vi "OAT Truncate Speed Profile.vi"(9 "window info":T2={"window type"=10, "window length"=2048} {"window type" items=["None"=0, "Hanning"=1, "Hamming"=2, "Blackman-Harris"=3, "Exact Blackman"=4, "Blackman"=5, "Flat Top"=6, "4 Term B-Harris"=7, "7 Term B-Harris"=8, "Low Sidelobe"=9, "Gaussian"=62]; "window length" min=0}, 10 "speed profile 2":T1 {"speed [RPM]" format="%.2f"; "time [s]" format="%.2f"}, 11 "order waveforms [EU]":waveform(dbl)[](array[waveform])) -> (2 "speed profile":T1 {"speed [RPM]" format="%.2f"; "time [s]" format="%.2f"})   [LabVIEW 2017, in "SoundVib_Resampling.lvlib"]
uses:
  <vilib>/addons/Sound and Vibration/Order Analysis/Resample Order Tracking/SoundVib_Resampling.lvlib
  <vilib>/addons/Sound and Vibration/Order Analysis/Ref Gabor Order Tracking/window information.ctl
  <vilib>/addons/Sound and Vibration/Order Analysis/Tach Process/SubVIs/speed profile.ctl
  <vilib>/addons/Sound and Vibration/Order Analysis/Tach Process/SoundVib_TachProcess.lvlib
  <vilib>/addons/Sound and Vibration/Order Analysis/Gabor Order Tracking/SoundVib_Gabor.lvlib
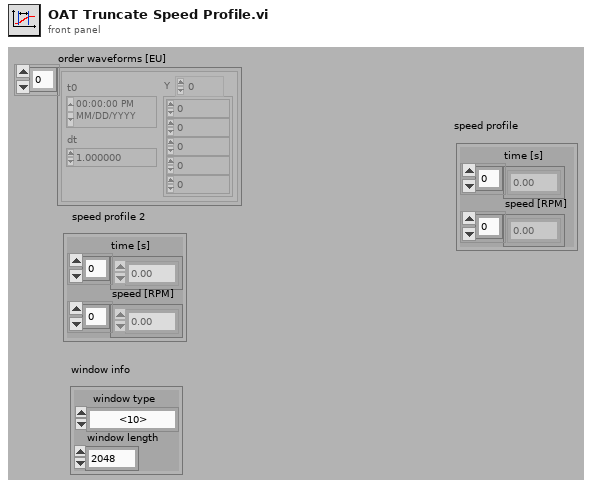
[diagram p1: front panel]
types:
  T1 = typedef "SoundVib_TachProcess.lvlib/speed profile.ctl" = cluster{"time [s]":dbl[], "speed [RPM]":dbl[]}
  T2 = typedef "SoundVib_Gabor.lvlib/window information.ctl" = cluster{"window type":u32, "window length":i32}
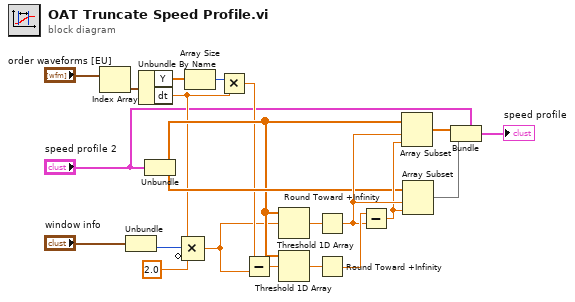
[diagram p0: block diagram]
diagram:
  n1 = Index Array(array="order waveforms [EU]") -> (element=w2:waveform(dbl))  [unwired: 1 in]
  n2 = Unbundle("window info") -> ("window length"=w11:i32)  [unwired: 1 out]
  n3 = Unbundle By Name(w2) -> ("Y"=w21:dbl[], "dt"=w8:dbl)
  n4 = Unbundle("speed profile 2") -> ("time [s]"=w12:dbl[], "speed [RPM]"=w17:dbl[])
  n5 = Compound Arithmetic op=MULTIPLY(w8, w11, invert 2.0) -> (w6:dbl)
  n6 = Array Size(array=w21) -> (size(s)=w9:i32)
  n7 = Multiply(x=w9, y=w8) -> (x*y=w7:dbl)
  n8 = Subtract(x=w7, y=w6) -> (x-y=w16:dbl)
  n9 = Threshold 1D Array(2:w6, 3:w12) -> (0:w14:dbl)  [unwired: 1 in]
  n10 = Threshold 1D Array(2:w16, 3:w12) -> (0:w15:dbl)  [unwired: 1 in]
  n11 = Round Toward +Infinity(x=w14) -> (ceil(x): smallest int >= x=w19:dbl)
  n12 = Round Toward +Infinity(x=w15) -> (ceil(x): smallest int >= x=w20:dbl)
  n13 = Subtract(x=w20, y=w19) -> (x-y=w18:dbl)
  n14 = Array Subset(array=w12, index=w19, length=w18) -> (w5:dbl[])
  n15 = Array Subset(array=w17, index=w19, length=w18) -> (w4:dbl[])
  n16 = Bundle(cluster="speed profile 2", "time [s]"=w5, "speed [RPM]"=w4) -> (→"speed profile":T1)
